vi "AddActorEnqueue.vi"(8 "error in (no error)":errorcluster, 9 "Actor's Enqueuer":refnum<class "Message Enqueuer.lvclass">, 10 "name":string, 11 "ActorMap in":refnum<class "ActorMap.lvclass">) -> (0 "error out":errorcluster, 3 "ActorMap out":refnum<class "ActorMap.lvclass">)   [LabVIEW 2020, in "ActorMap.lvclass"]
uses:
  ActorMap.lvclass
  <vilib>/ActorFramework/Message Enqueuer/Message Enqueuer.lvclass
  ActorMap.lvclass/ActorMap.ctl
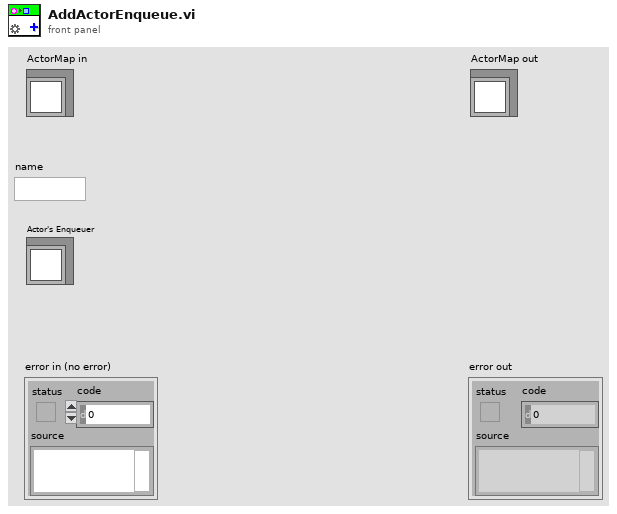
[diagram p1: front panel]
types:
  T1 = map{string, refnum<class "Message Enqueuer.lvclass">}
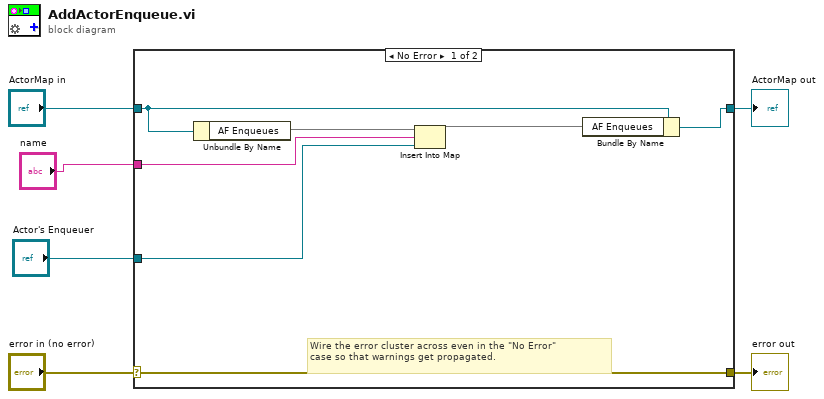
[diagram p0: block diagram]
diagram:
  n1 = case shown="No Error" "error in (no error)" {
    selector: "error in (no error)" -> [w13 w15]
    tunnel: [w13 w15] -> w5
    tunnel: [w7 w14] -> w3
    tunnel: "ActorMap in" -> [w9 w14]
    tunnel: "Actor's Enqueuer" -> [w10 _]
    tunnel: "name" -> [w11 _]
    frame No Error {
      # "Wire the error cluster across even in the \"No Error\"\ncase so that warnings get propagated."
      n2 = Unbundle By Name(w9) -> ("AF Enqueues"=w12:T1)
      n3 = Insert Into Map(map in=w12, key=w11, value=w10) -> (map out=w8:T1)  [unwired: 2 out]
      n4 = Bundle By Name(cluster=w9, "AF Enqueues"=w8) -> (w7:refnum<class "ActorMap.lvclass">)
    }
    frame Error {
    }
  }
  "error out" <- w5
  "ActorMap out" <- w3
